vi "Neos.vi"() -> ()   [LabVIEW 2026]
panel:
  out "Degrade Arriba":u32(colorbox)
  out "Degrade Abajo":u32(colorbox)
  in  "Retardo":u32=30
  in  "VISA resource name":refnum<visa-resource-name>
  in  "Seleccion de color":u32(colorbox)
  in  "Stop Button 2":bool
  # "Demo Degradado con Neopixeles"
  # "Degradado animado que baja y sube la intensidad del color seleccionado en las Neopixeles"
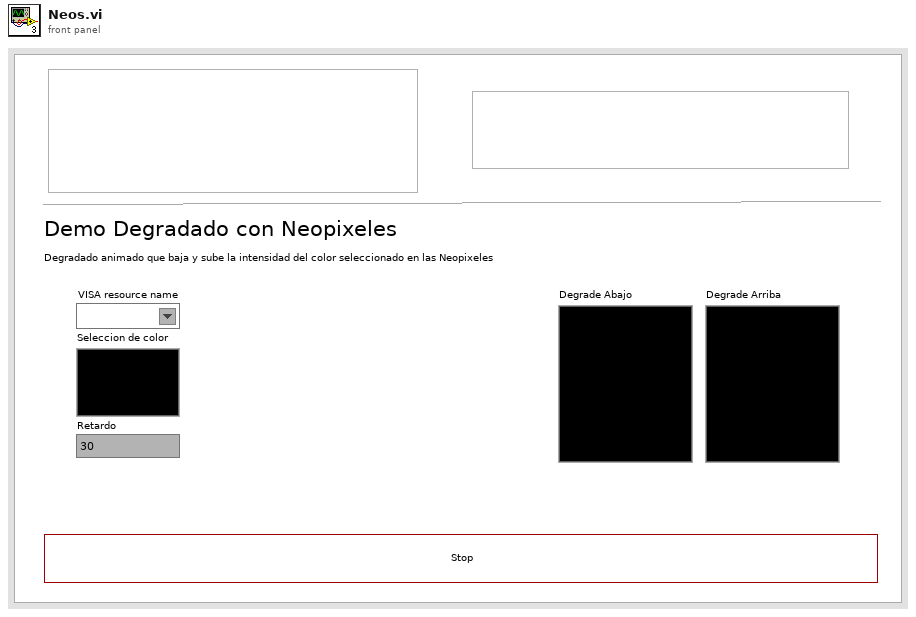
[diagram p1: front panel]
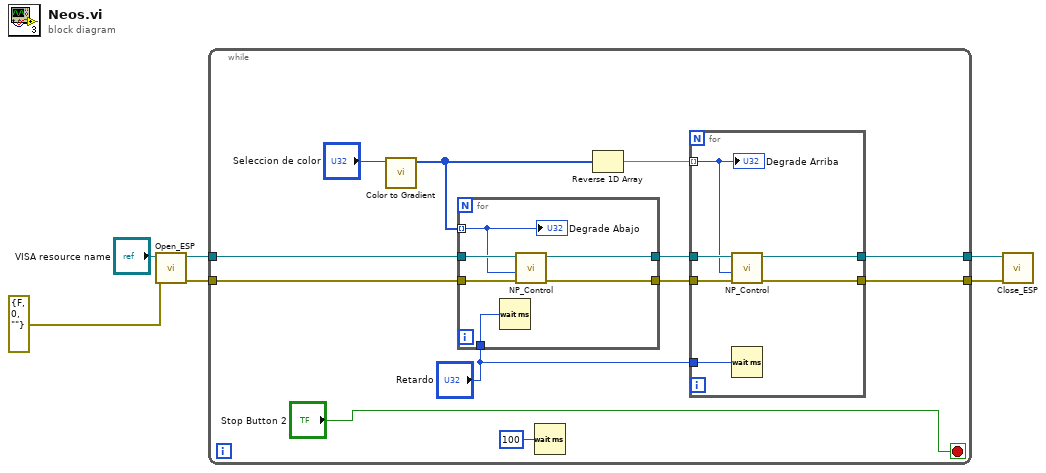
[diagram p0: block diagram]
diagram:
  n1 = call "Open_ESP.vi"("error in (no error)"=errorcluster {"status"=FALSE, "code"=0, "source"=""}, "VISA resource name"="VISA resource name") -> ("error out"=w3:errorcluster, "VISA resource name out"=w5:refnum<visa-resource-name>)  [unwired: 8 in]
  n2 = while {
    tunnel: w5 -> [w16]
    tunnel: [w11] -> w2
    tunnel: w3 -> [w15]
    tunnel: [w12] -> w4
    stop <- "Stop Button 2" stop-if-true
    n3 = call "Color to Gradient.vi"("Color Box"="Seleccion de color") -> ("Color Gradient"=w9:u32[])  [unwired: 7 in, 1 out]
    n4 = for {
      tunnel: w9 -> [w28] mode=indexing
      tunnel: w16 -> [w30]
      tunnel: [w29] -> w14
      tunnel: w15 -> [w27]
      tunnel: [w26] -> w13
      tunnel: "Retardo" -> [w25]
      n5 = Wait (ms)(milliseconds to wait=w25) -> ()  [unwired: 1 out]
      n6 = call "NP_Control.vi"("error in (no error)"=w27, "Color Box"=w28, "VISA resource name"=w30) -> ("error out"=w26:errorcluster, "VISA resource name out"=w29:refnum<visa-resource-name>)  [unwired: 7 in]
      "Degrade Abajo" <- w28
    }
    n7 = Wait (ms)(milliseconds to wait=u32 100) -> ()  [unwired: 1 out]
    n8 = Reverse 1D Array(array=w9) -> (reversed array=w10:u32[])
    n9 = for {
      tunnel: w10 -> [w22] mode=indexing
      tunnel: w14 -> [w24]
      tunnel: [w23] -> w11
      tunnel: w13 -> [w21]
      tunnel: [w20] -> w12
      tunnel: "Retardo" -> [w19]
      n10 = call "NP_Control.vi"("error in (no error)"=w21, "Color Box"=w22, "VISA resource name"=w24) -> ("error out"=w20:errorcluster, "VISA resource name out"=w23:refnum<visa-resource-name>)  [unwired: 7 in]
      n11 = Wait (ms)(milliseconds to wait=w19) -> ()  [unwired: 1 out]
      "Degrade Arriba" <- w22
    }
  }
  n12 = call "Close_ESP.vi"("error in (no error)"=w4, "VISA resource name"=w2) -> ()  [unwired: 9 in, 1 out]
